vi "Initialize BPMeaurement.vi"(2 "error in (no error)":errorcluster, 3 "Heart Rate Params":T1={"Heart Rates"=[], "Peak Pressures"=[], "Peak Amplitudes"=[], "History Length"=20, "Last  Slope"=20.0, "filtered history"=[], "raw history"=[], "Pulse"=FALSE, "Heart Rate Timer"=0, "Iteration"=0, "Pressure of Valley"=0.0, "Slope Log"=[], "Signal Segment"=refnum, "Acquisition Graph"=refnum, "This VI"=refnum, "Name"=""}) -> (0 "error out":errorcluster, 1 "Heart Rate Params 2":T1)   [LabVIEW 2017]
doc: "[Covers: SoftwareReq1]"
uses:
  Custom Controls/Heart Rate Parameters.ctl
panel:
  # "This VI demonstrates several failed tests that VI Analyzer shoudl catch, including overlapping objects and non-standard connector panes"
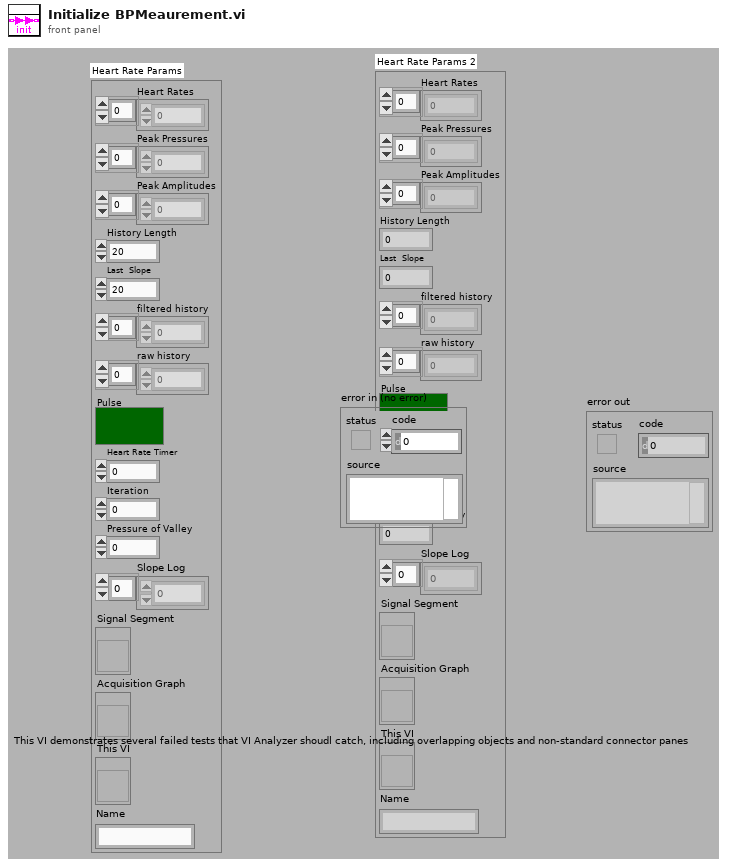
[diagram p1: front panel]
types:
  T1 = typedef "Heart Rate Parameters.ctl" = cluster{"Heart Rates":dbl[], "Peak Pressures":dbl[], "Peak Amplitudes":dbl[], "History Length":i32, "Last  Slope":dbl, "filtered history":dbl[], "raw history":dbl[], "Pulse":bool, "Heart Rate Timer":i32, "Iteration":u32, "Pressure of Valley":dbl, "Slope Log":dbl[], "Signal Segment":refnum<vi>, "Acquisition Graph":refnum<vi>, "This VI":refnum<vi>, "Name":string}
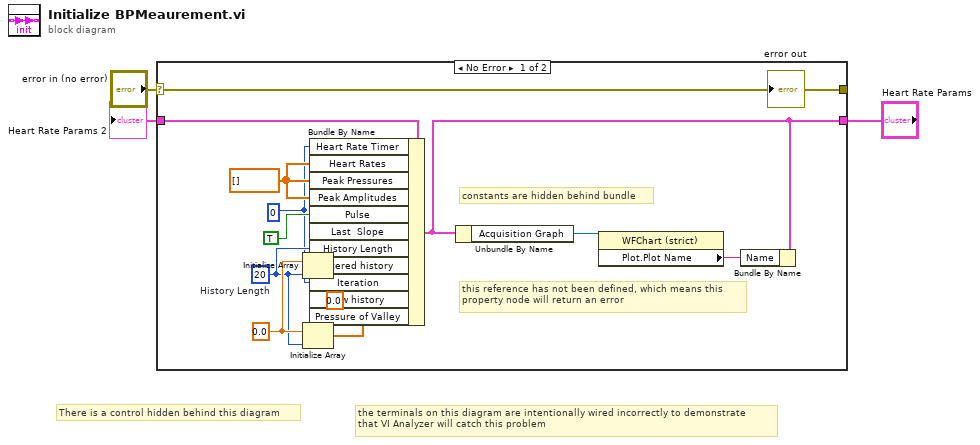
[diagram p0: block diagram]
diagram:
  # "There is a control hidden behind this diagram"
  # "the terminals on this diagram are intentionally wired incorrectly to demonstrate\nthat VI Analyzer will catch this problem"
  n1 = case shown="No Error" "error in (no error)" {
    selector: "error in (no error)" -> [w9 w18]
    tunnel: [w9 w18] -> w4
    tunnel: [w8 _] -> w2
    tunnel: "Heart Rate Params" -> [w6 _]
    frame No Error {
      w11 = 0.0 ("Pressure of Valley")
      w10 = 0 ("Heart Rate Timer")
      w14 = 20  # History Length
      w16 = dbl[] []
      w17 = 0.0 ("element")
      # "this reference has not been defined, which means this\nproperty node will return an error"
      # "constants are hidden behind bundle"
      n2 = Initialize Array(w17, w14) -> (w13:dbl[])
      n3 = Initialize Array(w17, w14) -> (w12:dbl[])
      n4 = Bundle By Name(cluster=w6, "Heart Rate Timer"=w10, "Heart Rates"=w16, "Peak Pressures"=w16, "Peak Amplitudes"=w16, "Pulse"=TRUE, "Last  Slope"=w11, "History Length"=w14, "filtered history"=w13, "Iteration"=w10, "raw history"=w12, "Pressure of Valley"=w11) -> (w8:T1)
      n5 = Unbundle By Name(w6) -> ("Acquisition Graph"=w7:refnum<vi>)
      n6 = property class="WFChart (strict)"(reference=w7) -> ("Plot.Plot Name"=w5:string)  [unwired: 1 in, 2 out]
      n7 = Bundle By Name(cluster=w6, "Name"=w5) -> ()  [unwired: 1 out]
    }
    frame Error {
    }
  }
  "error out" <- w4
  "Heart Rate Params 2" <- w2
